vi "Set Global Attribute.vi"(8 "Error In":errorcluster, 9 "Delete (F)":bool, 10 "Value":variant, 11 "Name":string) -> (0 "Error Out":errorcluster, 3 "dup Name":string)   [LabVIEW 2013, in "TS.lvlib"]
doc: "Non-reentrant."
uses:
  TS.lvlib
  Variant Global.vi
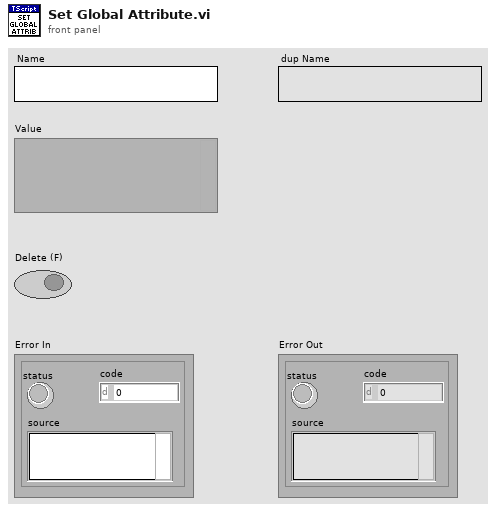
[diagram p1: front panel]
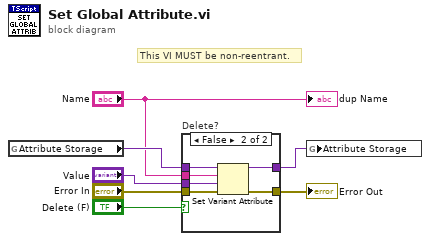
[diagram p0: block diagram]
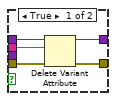
[diagram p2: hidden frame]
diagram:
  # "This VI MUST be non-reentrant."
  n1 = global read "Variant Global.vi" "Attribute Storage"() -> (w7:variant)
  n2 = case "Delete?" shown="False" "Delete (F)" {
    tunnel: w7 -> [w8 w18]
    tunnel: "Value" -> [_ w17]
    tunnel: "Error In" -> [w12 w16]
    tunnel: [w11 w15] -> w4
    tunnel: [w10 w14] -> w3
    tunnel: "Name" -> [w9 w13]
    frame True {
      n3 = Delete Variant Attribute(4:w12, 6:w9, 7:w8) -> (0:w11:errorcluster, 3:w10:variant)  [unwired: 1 out]
    }
    frame False {
      n4 = Set Variant Attribute(Variant=w18, name=w13, value=w17, error in=w16) -> (Variant out=w14:variant, error out=w15:errorcluster)  [unwired: 1 out]
    }
  }
  "Error Out" <- w4
  n5 = global write "Variant Global.vi" "Attribute Storage"(w3) -> ()
  "dup Name" <- "Name"
